vi "program seq..vi"(6 "IOList":T3, 7 "Cluster data":T5, 11 "Filepath":path=path "E:/My Project/2018-2019/Under development/Minda Ind. Switch -ID 144-145/Project/data/trail pro -12.txt") -> (0 "Error Out":errorcluster)   [LabVIEW 2015]
uses:
  Control PB/Active.ctl
  Control PB/deactive.ctl
  Control PB/output control.ctl
  Control PB/input control.ctl
  Control PB/timer.ctl
  Control PB/Remove list.ctl
  Control Button/Exit.ctl
  Control PB/Add_s.ctl
  Control PB/Delete_.ctl
  Control Button/Save.ctl
  Control PB/motor.ctl
  Control PB/Camera.ctl
  Control PB/Barcode.ctl
  Galobal variable_TI.vi
panel:
  out "Step List 4":string[](array[string])
  out "Step List 3":string[](array[string])
  in  "Barcode":T1
  in  "Camera":T2
  out "x <= y?":bool
  out "Cancel":bool
  out "Step List 2":string[](array[string])
  out "Pokayoka Result":cluster{"Sensor Name":string, "Boolean":bool}[](array[cluster])
  in  "Feed Back Channel":i32[](listbox)=[0]
  out "Input":bool[](array[boolean])
  out "Feature List (Out) 2":T4(array[cluster])
  out "error out 2":errorcluster
  in  "Control":bool
  out "Station No":string
  out "Model Name":string
  out "Machine Name":string
  in  "Motor":T6
  in  "Feature List":i32(listbox) caption="Steps List"
  in  "Deletefeature list":T7
  in  "Add feature list":T8
  in  "Deactive":T9
  in  "Active":T10
  in  "Program step":i32(listbox)
  in  "Remove Step":T11
  in  "Wait Time":u32=100 caption="Timer(ms)" max=600000 step=1
  in  "Timer":T12
  in  "Save":T13
  in  "stop":T14
  in  "op Add":T15
  in  "Input Add":T16
  out "Step List":string[](array[string])
  out "output cluster":T17
  in  "Analog":bool
  in  "Analog Input":i32[](listbox)=[0]
  in  "Control Channel":i32[](listbox)=[7]
  in  "Steps":T18(array[cluster])
  in  "Program mode":string="Data"
  out "error out":errorcluster
  out "Feature List (Out)":T19(array[cluster])
  # "Program Sequence Window"
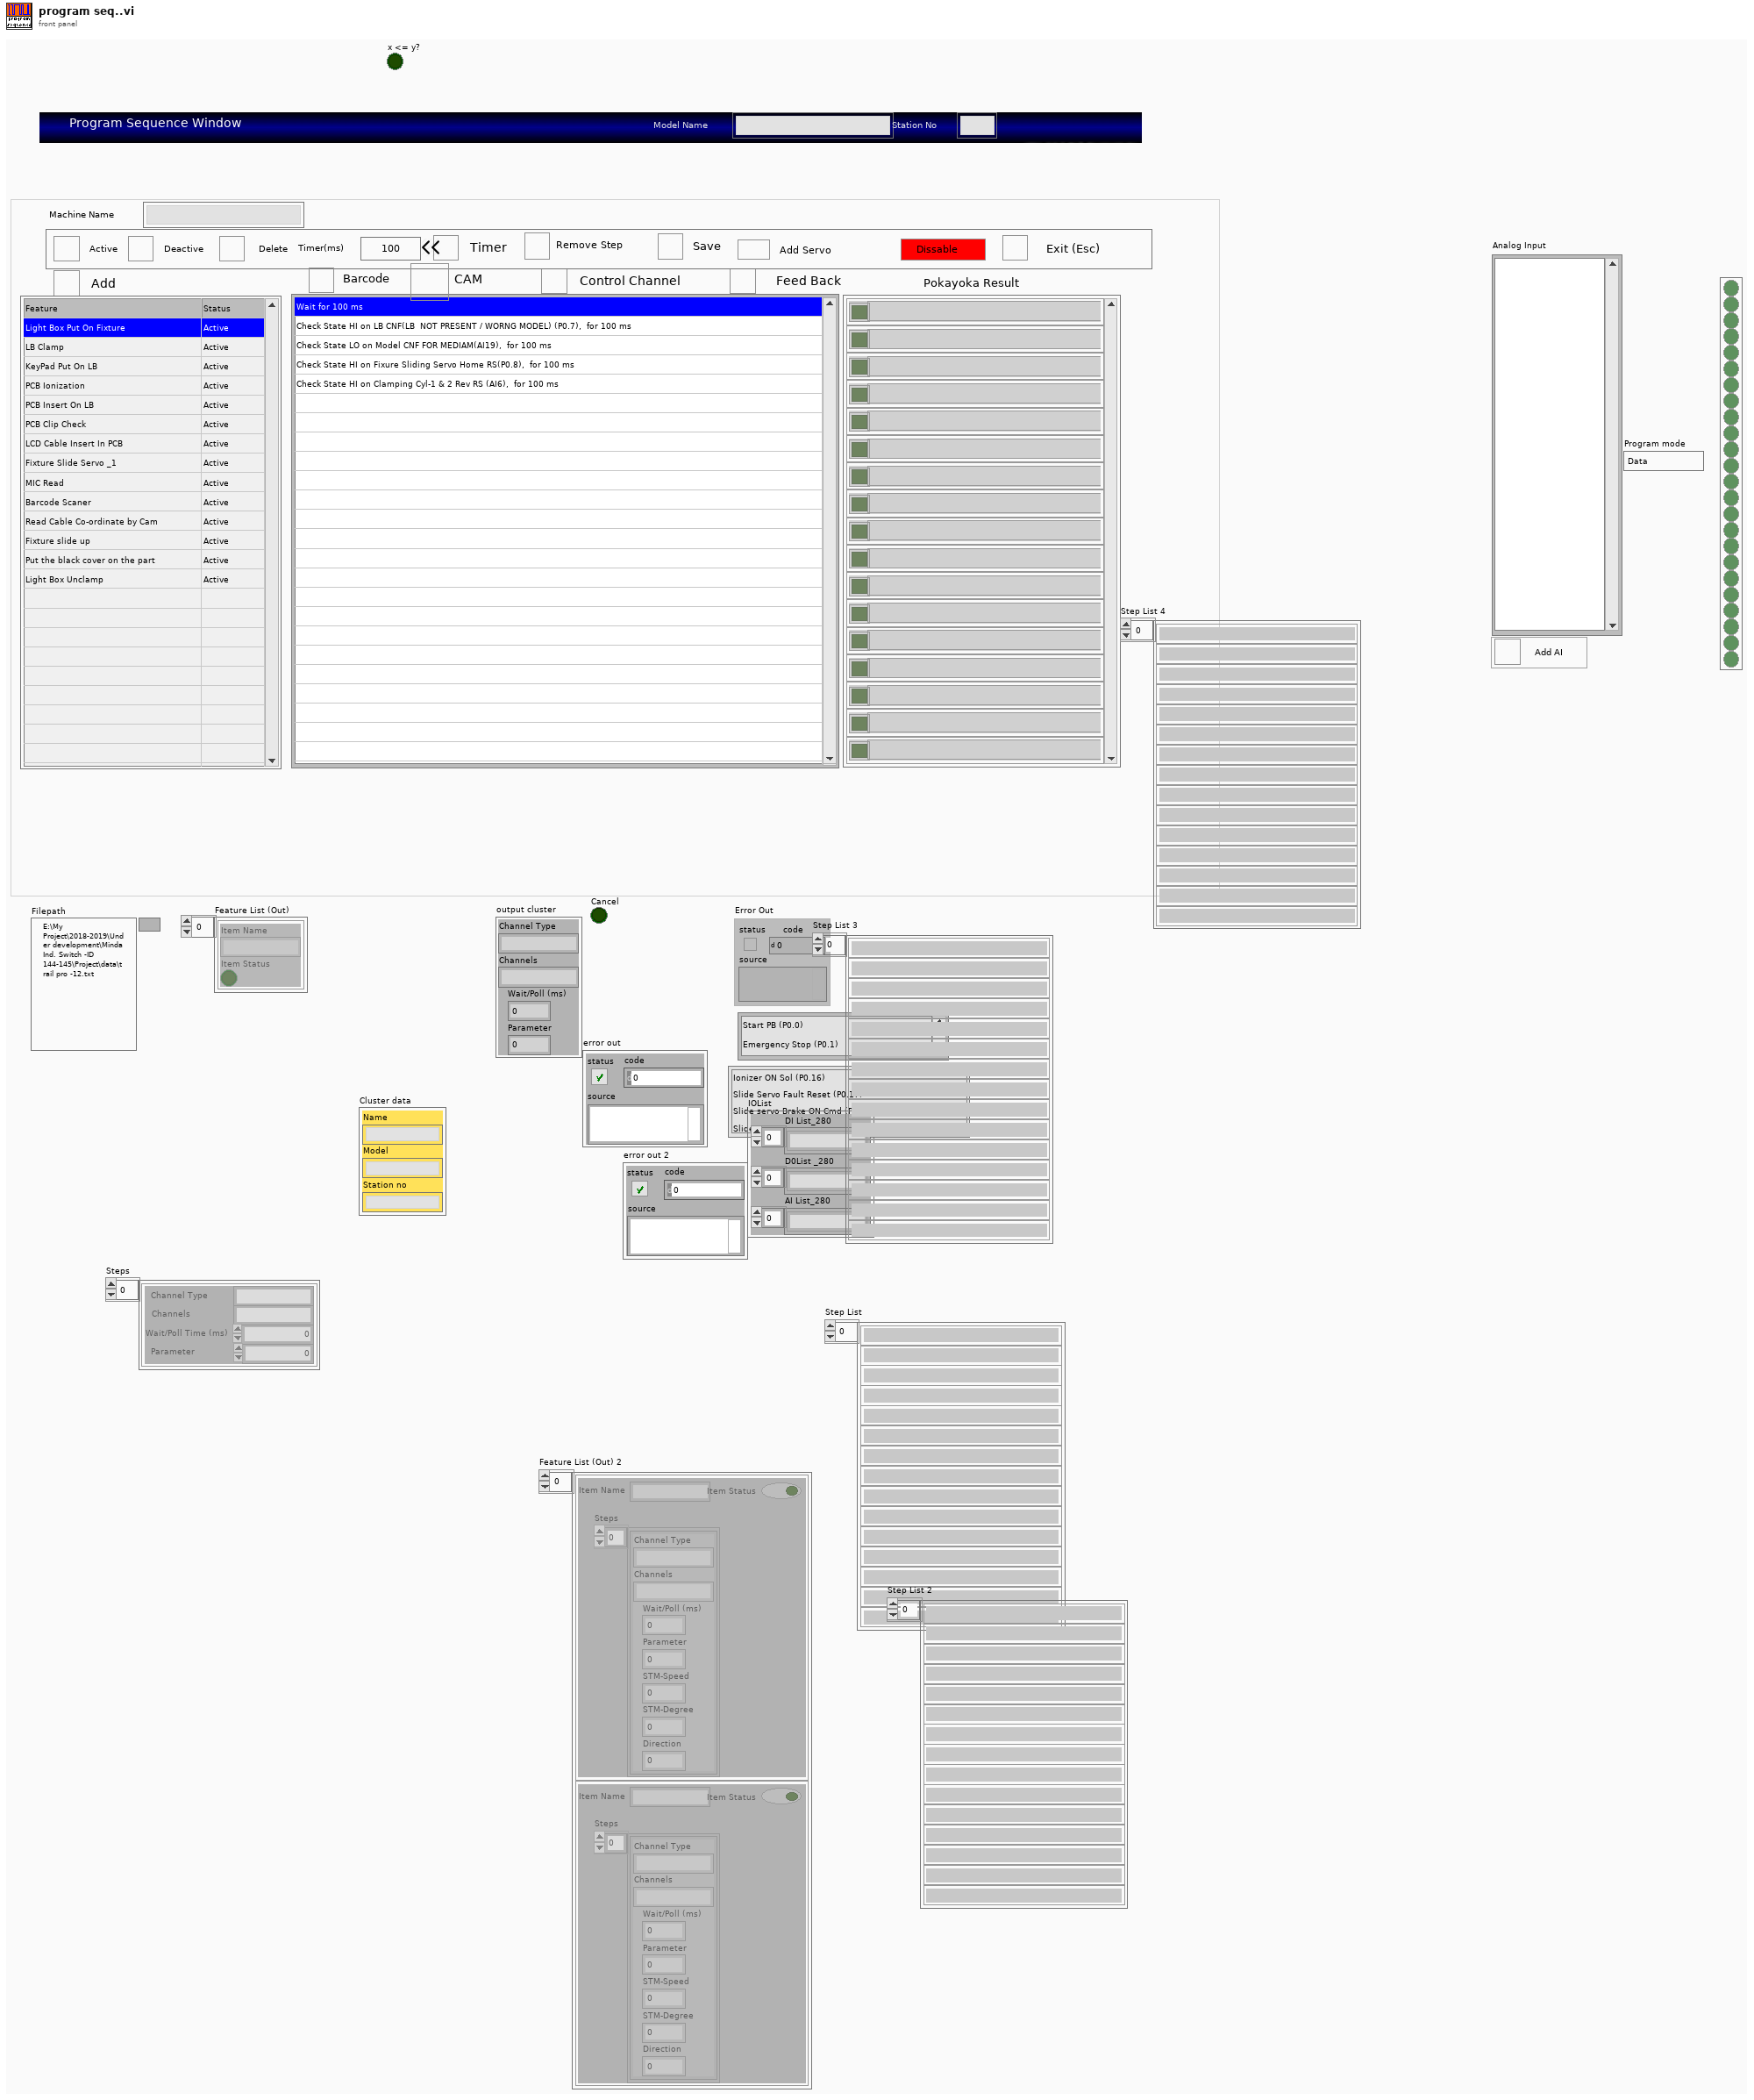
[diagram p1: front panel]
types:
  T1 = typedef "Barcode.ctl" = bool
  T2 = typedef "Camera.ctl" = bool
  T3 = cluster{"DI List_280":string[], "D0List _280":string[], "AI List_280":string[]}
  T4 = cluster{"Item Name":string, "Item Status":bool, "Steps":cluster{"Channel Type":string, "Channels":string, "Wait/Poll (ms)":u32, "Parameter":u8, "STM-Speed":i32, "STM-Degree":u32, "Direction":u8}[]}[]
  T5 = cluster{"Name":string, "Model":string, "Station no":string}
  T6 = typedef "motor.ctl" = bool
  T7 = typedef "Delete_.ctl" = bool
  T8 = typedef "Add_s.ctl" = bool
  T9 = typedef "deactive.ctl" = bool
  T10 = typedef "Active.ctl" = bool
  T11 = typedef "Remove list.ctl" = bool
  T12 = typedef "timer.ctl" = bool
  T13 = typedef "Save.ctl" = bool
  T14 = typedef "Exit.ctl" = bool
  T15 = typedef "output control.ctl" = bool
  T16 = typedef "input control.ctl" = bool
  T17 = cluster{"Channel Type":string, "Channels":string, "Wait/Poll (ms)":u32, "Parameter":u8}
  T18 = cluster{"Channel Type":string, "Channels":string, "Wait/Poll Time (ms)":u32, "Parameter":u8}[]
  T19 = cluster{"Item Name":string, "Item Status":bool}[]
  T20 = cluster{"Channel Type":string, "Channels":string, "Wait/Poll (ms)":u32, "Parameter":u8, "STM-Speed":i32, "STM-Degree":i32, "Direction":u8}
  T21 = cluster{"Item Name":string, "Item Status":bool, "Steps":cluster{"Channel Type":string, "Channels":string, "Wait/Poll (ms)":u32, "Parameter":u8, "STM-Speed":i32, "STM-Degree":u32, "Direction":u8}[]}
  T22 = cluster{"Channel Type":string, "Channels":string, "Wait/Poll (ms)":u32, "Parameter":u8, "STM-Speed":i32, "STM-Degree":u32, "Direction":u8}[]
  T23 = cluster{"Item Name":string, "Active":T10, "Steps":cluster{"Channel Type":string, "Channels":string, "Wait/Poll (ms)":u32, "Parameter":u8, "STM-Speed":i32, "STM-Degree":u32, "Direction":u8}[]}
  T24 = cluster{"Channel Type":string, "Channels":string, "Wait/Poll (ms)":u32, "Parameter":u8, "STM-Speed":i32, "STM-Degree":i32, "Direction":u8}[]
  T25 = cluster{"Feature name ":string, bool, cluster{"Channel Type":string, "Channels":string, "Wait/Poll (ms)":u32, "Parameter":u8, "STM-Speed":i32, "STM-Degree":i32, "Direction":u8}[]}
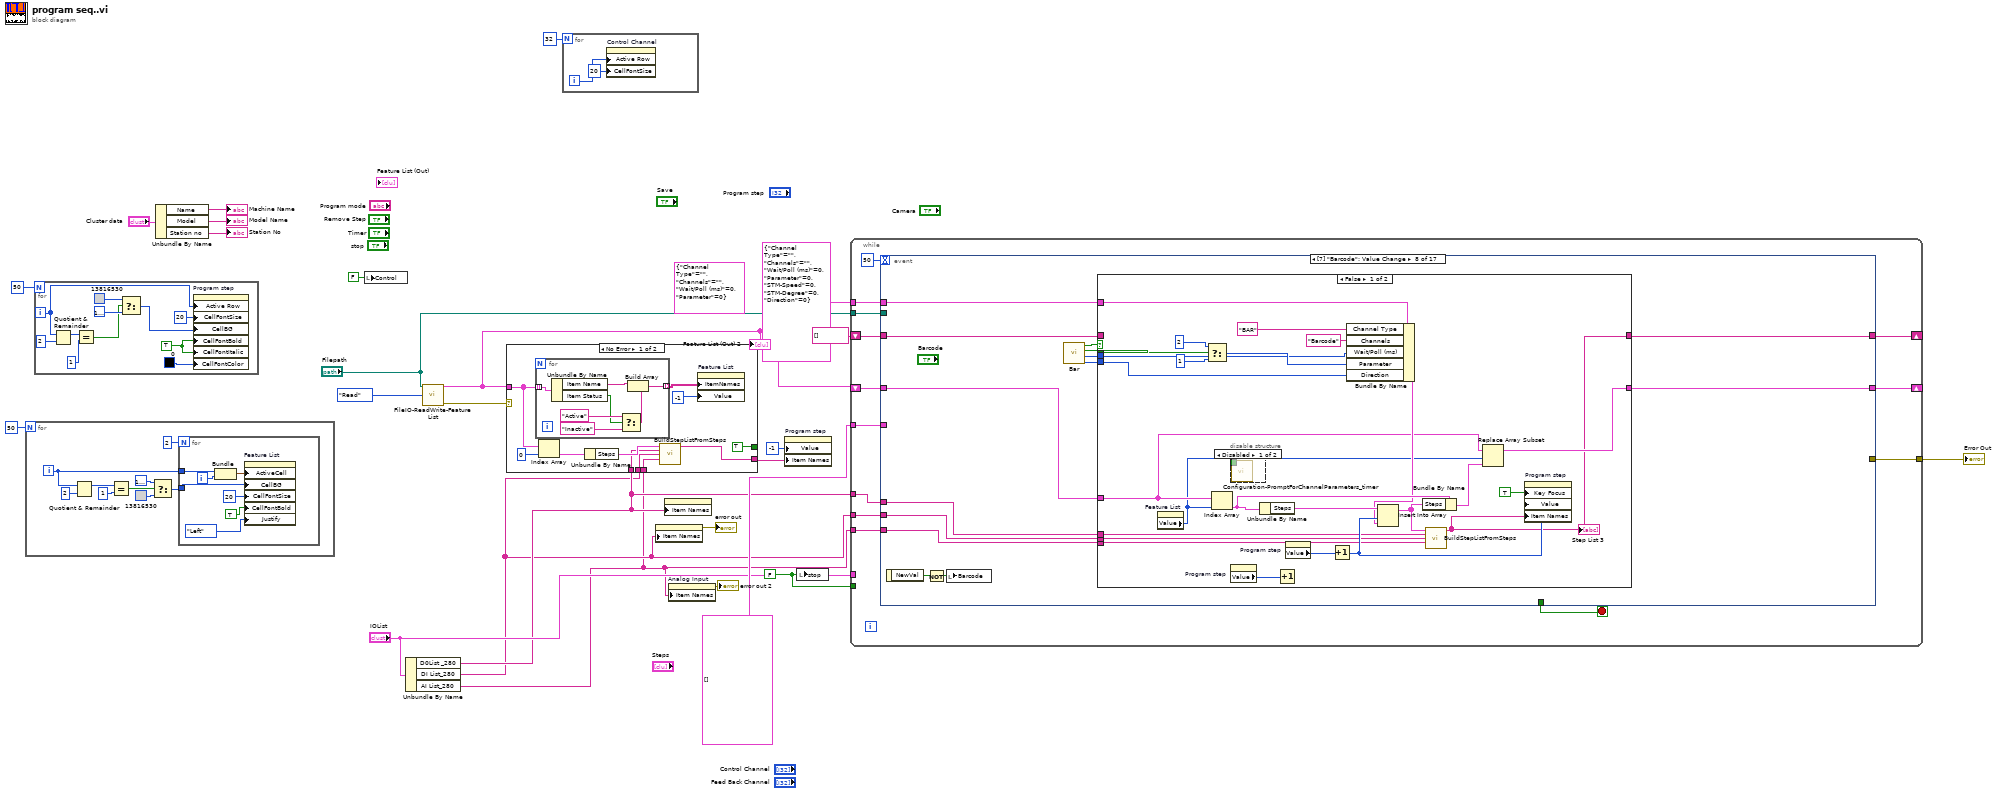
[diagram p0: block diagram]
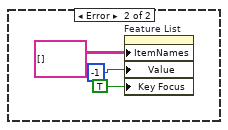
[diagram p2: hidden frame]
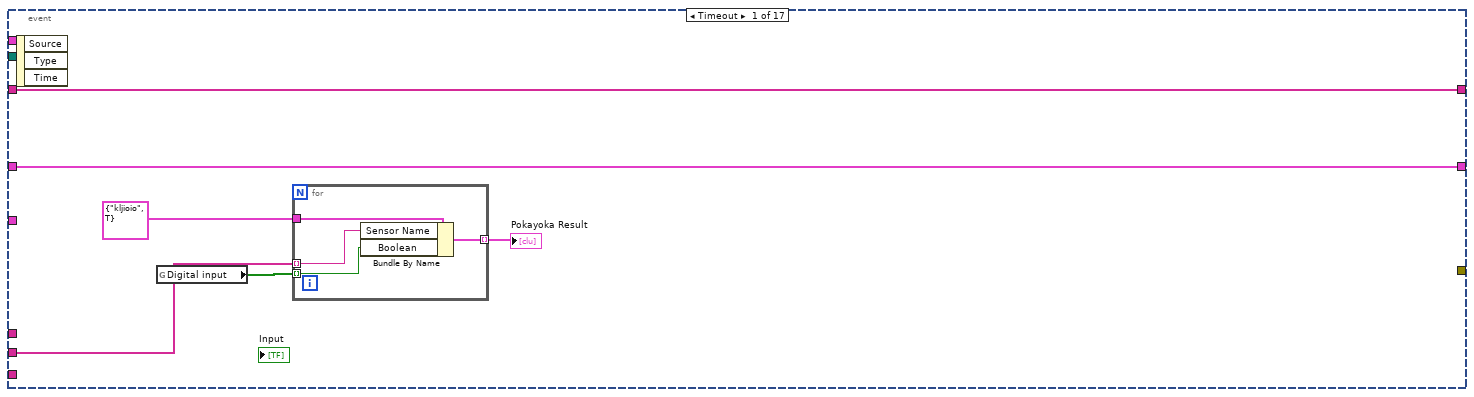
[diagram p3: hidden frame]
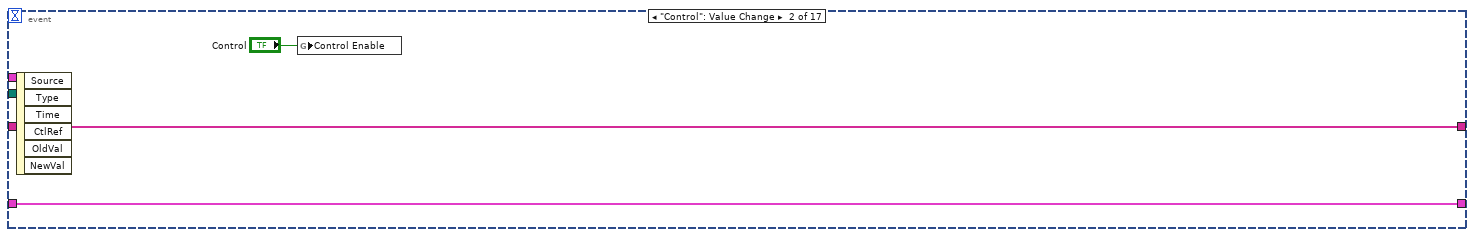
[diagram p4: hidden frame]
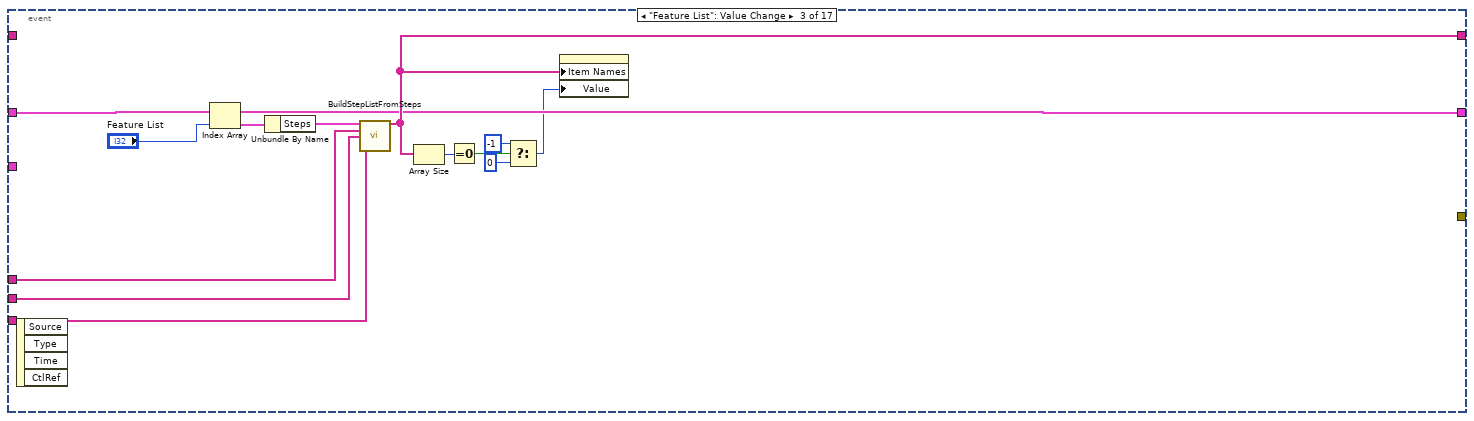
[diagram p5: hidden frame]
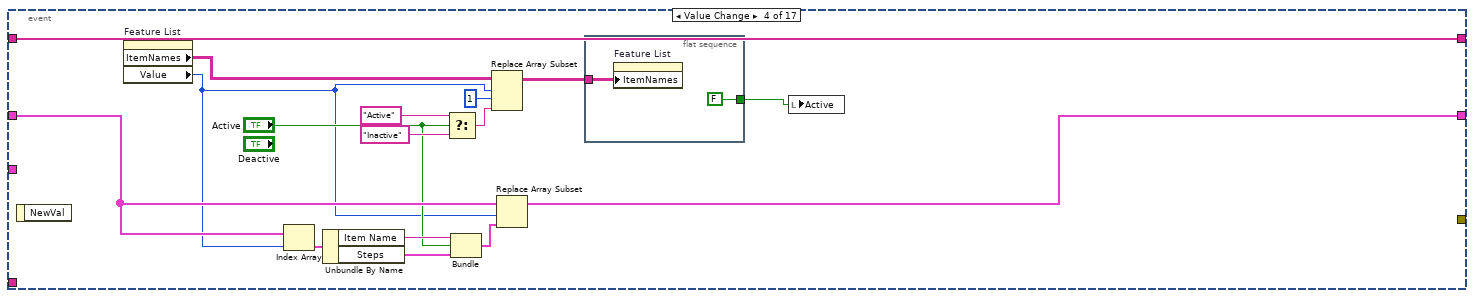
[diagram p6: hidden frame]
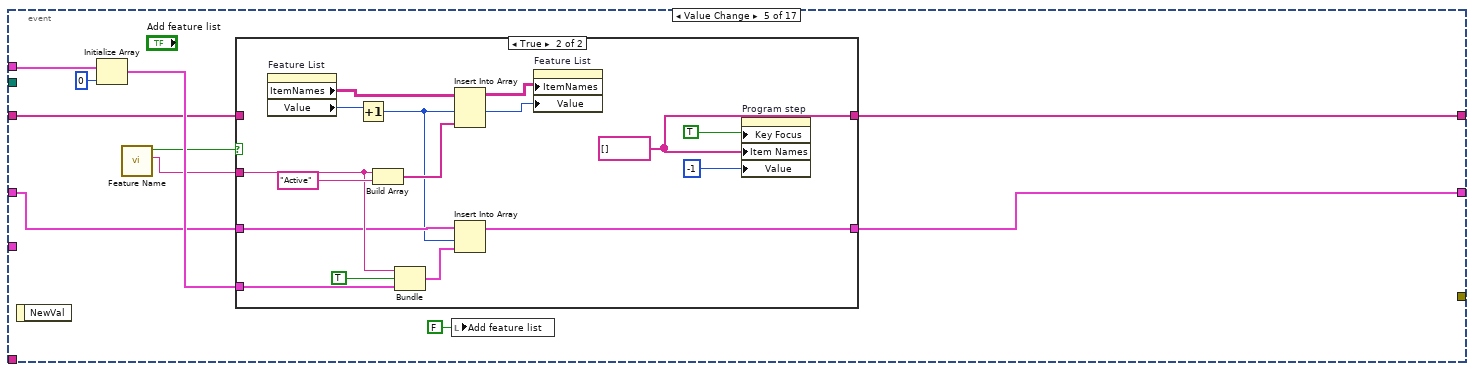
[diagram p7: hidden frame]
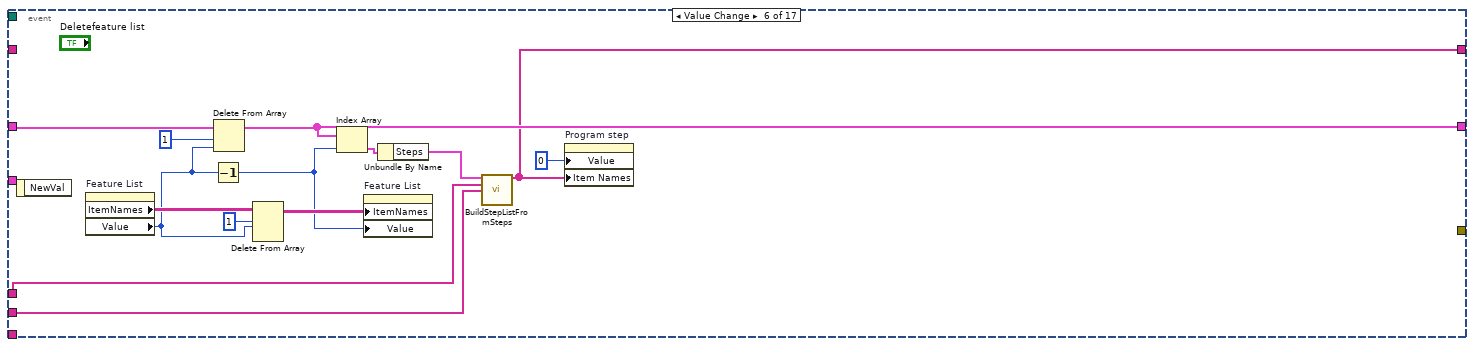
[diagram p9: hidden frame]
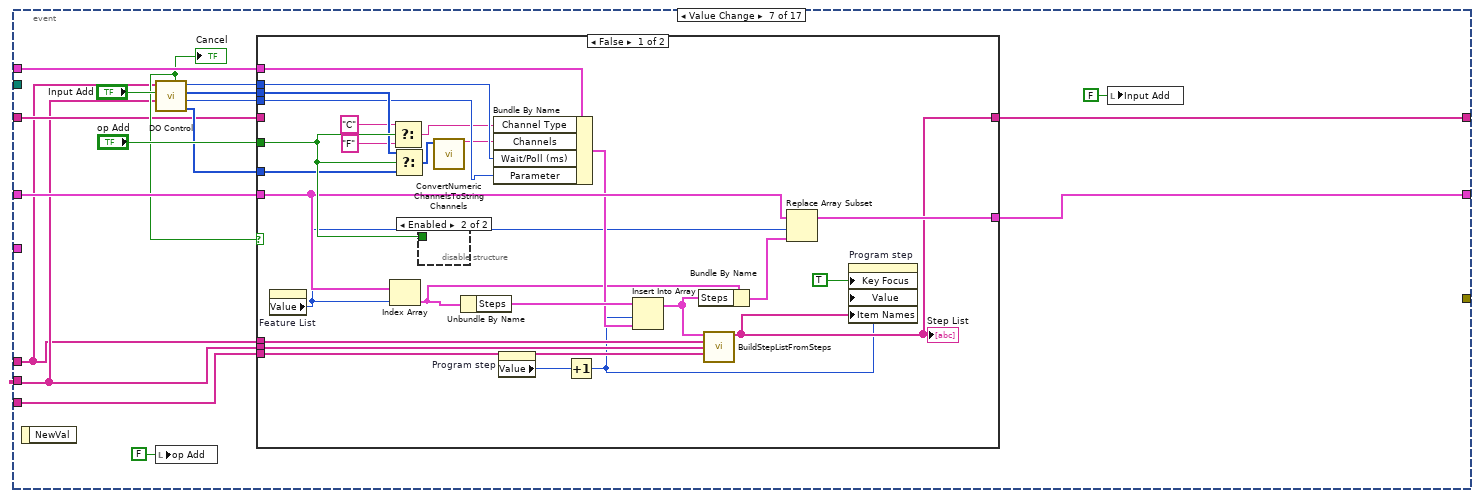
[diagram p10: hidden frame]
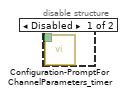
[diagram p11: hidden frame]
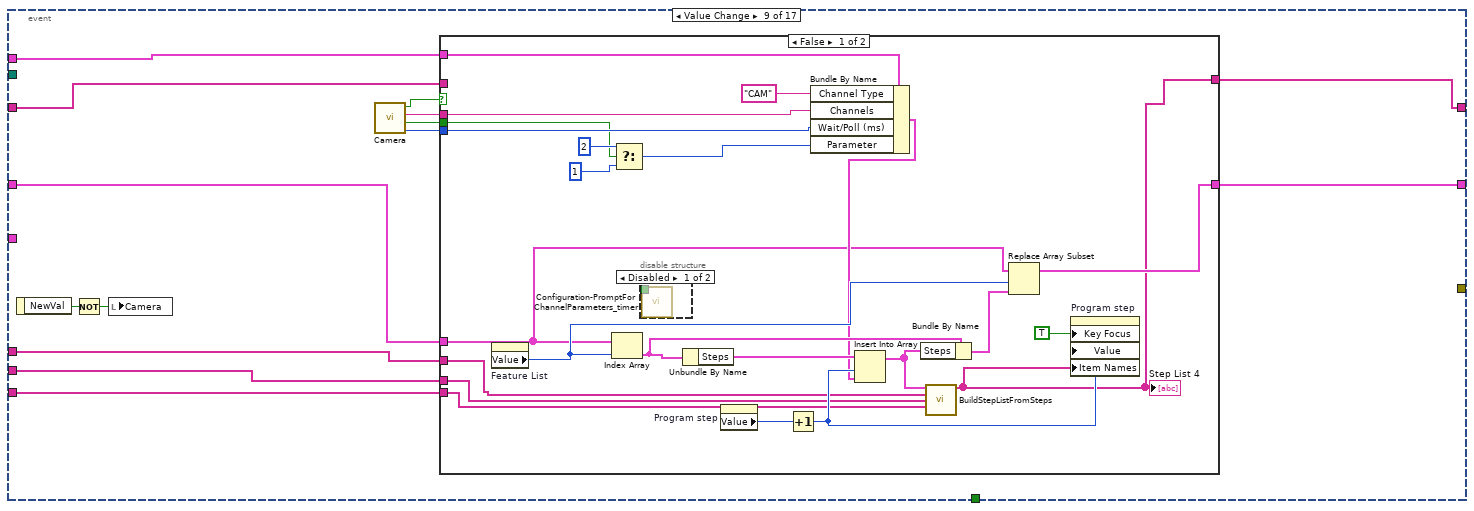
[diagram p15: hidden frame]
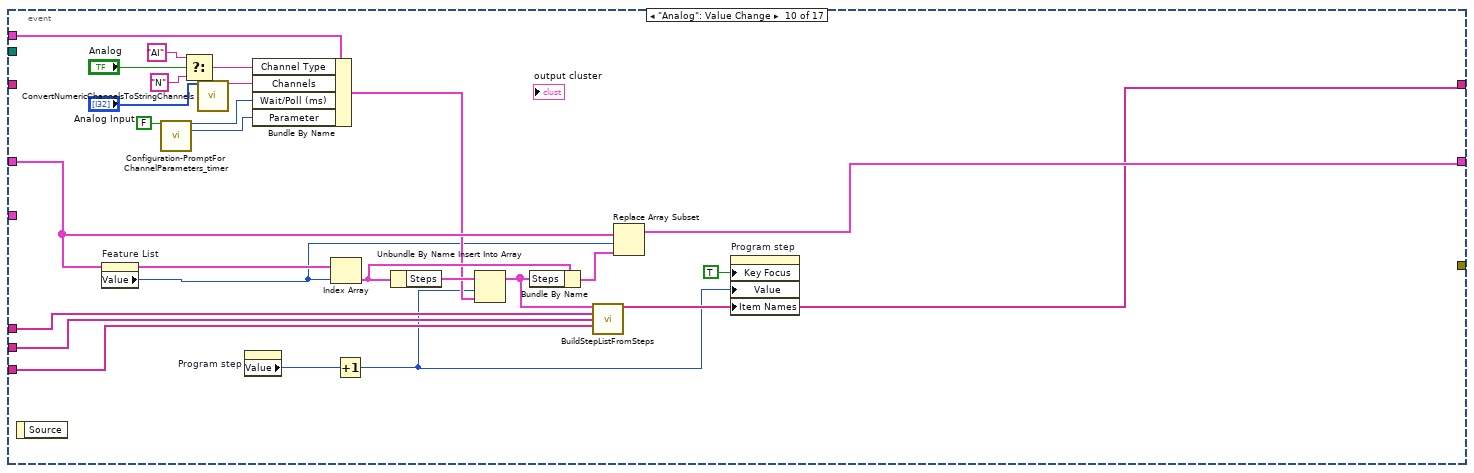
[diagram p18: hidden frame]
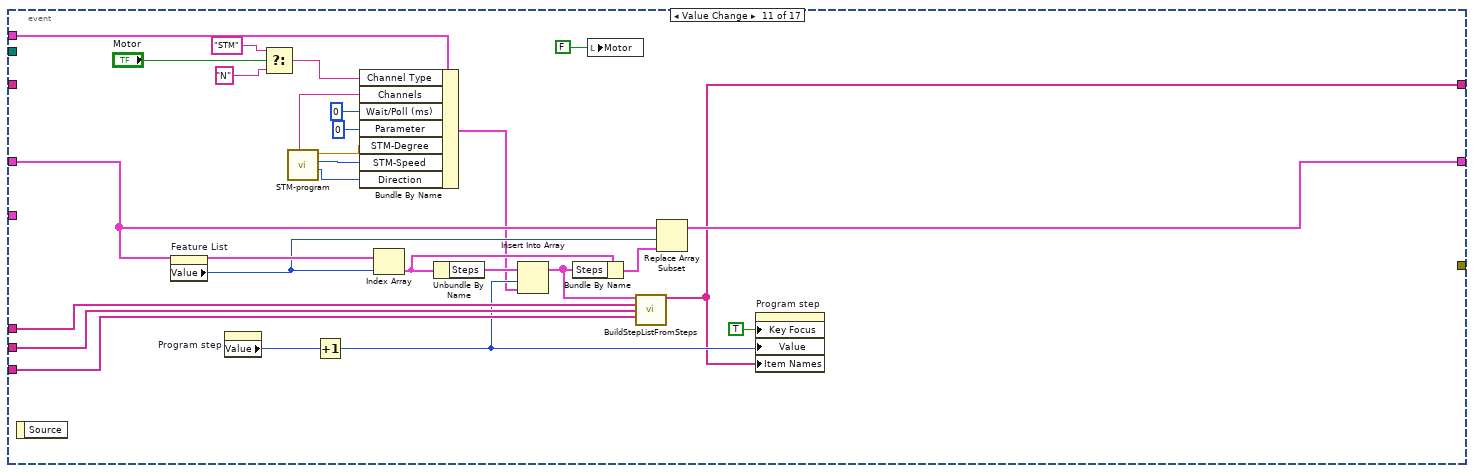
[diagram p19: hidden frame]
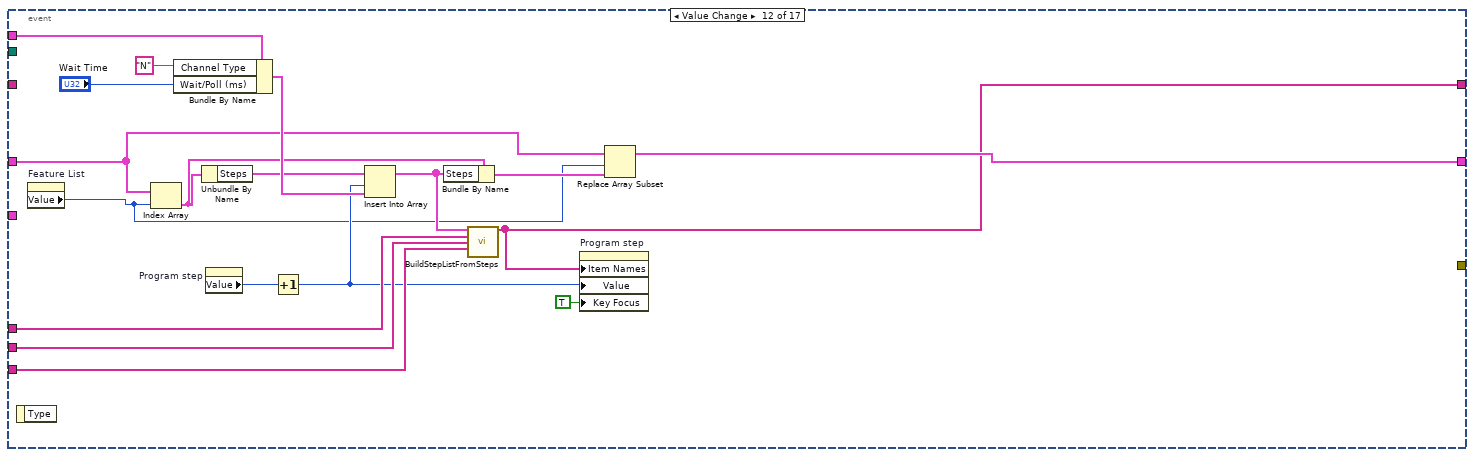
[diagram p20: hidden frame]
diagram:
  w8 = FALSE ("stop")
  (unwired) T17 {"Channel Type"="", "Channels"="", "Wait/Poll (ms)"=0, "Parameter"=0} ("Step")
  n1 = for {
    N: 50 -> [_]
    i -> [w33]
    n2 = Quotient & Remainder(x=w33, y=2) -> (x-y*floor(x/y)=w31:i32)  [unwired: 1 out]
    n3 = Equal?(x=w31, y=1) -> (x = y?=w29:bool)
    n4 = Select(t=u32 16777225 ("Color Box"), s=w29, f=u32 13816530 ("Color Box")) -> (s? t:f=w26:u32)
    n5 = for {
      N: 2 -> [_]
      tunnel: w33 -> [w41]
      tunnel: w26 -> [w38]
      i -> [w40]
      n6 = Bundle(w41, w40) -> (w39:cluster{i32, i32})  [unwired: 1 in]
      n7 = property on="Feature List" class="MCListbox (strict)"("ActiveCell"=w39, "CellBG"=w38, "CellFontSize"=u32 20 ("Active Cell:Cell Font:Size"), "CellFontBold"=TRUE ("Active Cell:Cell Font:Bold"), "Justify"=enum16{"Left", "Center", "Right"}."Left" ("Active Cell:Cell Justification")) -> ()  [unwired: 2 in, 2 out]
    }
  }
  n8 = for {
    N: 50 -> [_]
    i -> [w46]
    w43 = TRUE
    n9 = Quotient & Remainder(x=w46, y=2) -> (x-y*floor(x/y)=w49:i32)  [unwired: 1 out]
    n10 = Equal?(x=w49, y=1) -> (x = y?=w47:bool)
    n11 = Select(t=u32 13816530 ("Color Box"), s=w47, f=u32 16777226 ("Color Box")) -> (s? t:f=w44:u32)
    n12 = property on="Program step" class="LstBox (strict)"("Active Row"=w46, "CellFontSize"=u32 20 ("Active Row:Cell Font:Size"), "CellBG"=w44, "CellFontBold"=w43, "CellFontItalic"=w43, "CellFontColor"=u32 0 ("Color Box")) -> ()  [unwired: 2 in, 2 out]
  }
  n13 = Unbundle By Name("Cluster data") -> ("Name"=→"Machine Name":string, "Model"=→"Model Name":string, "Station no"=→"Station No":string)
  n14 = local write "Control"(FALSE ("Control")) -> ()
  n15 = Unbundle By Name("IOList") -> ("D0List _280"=w4:string[], "DI List_280"=w3:string[], "AI List_280"=w2:string[])
  n16 = call "FileIO-ReadWrite-FeatureList.vi"("Filepath"="Filepath", "Read/Write"=enum16{"Read", "Write"}."Read") -> ("Feature List (Out)"=w16:T4, "Error Out"=w20:errorcluster)  [unwired: 12 in]
  "Feature List (Out) 2" <- w16
  n17 = case shown="No Error" w20 {
    tunnel: w16 -> [w63 _]
    tunnel: w4 -> [w59 _]
    tunnel: w3 -> [w58 _]
    tunnel: w2 -> [w57 _]
    tunnel: [w56 _] -> w19
    tunnel: [TRUE ("Key Focus") _] -> _
    frame No Error {
      n18 = for {
        tunnel: w63 -> [w70] mode=indexing
        tunnel: [w64] -> w54 mode=indexing
        n19 = Unbundle By Name(w70) -> ("Item Name"=w66:string, "Item Status"=w67:bool)
        n20 = Select(t="Active", s=w67, f="Inactive") -> (s? t:f=w65:string)
        n21 = Build Array(w66, w65) -> (w64:string[])
      }
      n22 = Index Array(array=w63, index=0) -> (element=w61:T21)
      n23 = Unbundle By Name(w61) -> ("Steps"=w60:T22)
      n24 = call "BuildStepListFromSteps.vi"("Steps"=w60, "Control Channels"=w59, "Feedback Channels"=w58, "AI"=w57) -> ("Step List"=w56:string[])  [unwired: 11 in]
      n25 = property on="Feature List" class="MCListbox (strict)"("ItemNames"=w54, "Value"=-1 ("Feautre list")) -> ()  [unwired: 2 in, 2 out]
    }
    frame Error {
      n26 = property on="Feature List" class="MCListbox (strict)"("ItemNames"=string[][] [] ("Item Names"), "Value"=-1 ("Feautre list"), "Key Focus"=TRUE) -> ()  [unwired: 2 in, 2 out]
    }
  }
  n27 = for {
    N: 32 -> [_]
    i -> [w75]
    n28 = property on="Control Channel" class="LstBox (strict)"("Active Row"=w75, "CellFontSize"=u32 20 ("Active Row:Cell Font:Size")) -> ()  [unwired: 2 in, 2 out]
  }
  n29 = property on="Feed Back Channel" class="LstBox (strict)"("Item Names"=w3) -> (error out=→"error out":errorcluster)  [unwired: 2 in, 1 out]
  n30 = property on="Control Channel" class="LstBox (strict)"("Item Names"=w4) -> ()  [unwired: 2 in, 2 out]
  n31 = property on="Analog Input" class="LstBox (strict)"("Item Names"=w2) -> (error out=→"error out 2":errorcluster)  [unwired: 2 in, 1 out]
  n32 = property on="Program step" class="LstBox (strict)"("Value"=-1 ("Step feautre list"), "Item Names"=w19) -> ()  [unwired: 2 in, 2 out]
  n33 = local write "stop"(w8) -> ()
  n34 = while {
    shift-right: [w86] -> _
    shift-left: w16 -> [w77]
    tunnel: T20 {"Channel Type"="", "Channels"="", "Wait/Poll (ms)"=0, "Parameter"=0, "STM-Speed"=0, "STM-Degree"=0, "Direction"=0} ("Step") -> [w87]
    shift-right: [w85] -> _
    shift-left: string[] [] ("Step List") -> [w84]
    tunnel: w4 -> [w83]
    tunnel: w3 -> [w82]
    tunnel: [w81] -> w23
    tunnel: w2 -> [w80]
    tunnel: T4 [] ("Feature List (Out) 2") -> [w79]
    tunnel: "Filepath" -> [w78]
    tunnel: w8 -> [_]
    tunnel: "IOList" -> [_]
    stop <- w88 stop-if-true
    n35 = event shown="[7] \"Barcode\": Value Change" {
      selector: _ -> [_ _ _ _ _ _ _ _ _ _ _ _ _ _ _ _ _]
      dyn-events: _ -> [_ _ _ _ _ _ _ _ _ _ _ _ _ _ _ _ _]
      timeout: 50 -> [_ _ _ _ _ _ _ _ _ _ _ _ _ _ _ _ _]
      tunnel: [_ _ _ _ _ _ _ _ _ _ _ _ _ _ TRUE ("stop") _ TRUE ("Discard?")] -> w88
      tunnel: w77 -> [w94 w100 w105 w122 w139 w171 w187 w228 w271 w311 w341 w362 w384 w393 w453 w475 w552]
      tunnel: w87 -> [_ _ _ _ w142 _ w190 w233 w275 w318 w346 w371 _ _ _ w476 _]
      tunnel: [w94 w100 w105 w120 w138 w170 w188 w227 w270 w306 w333 w361 w383 w395 w453 w471 w552] -> w86
      tunnel: [w93 w101 w108 w119 w135 w165 w186 w226 w269 w305 w332 w358 w378 w410 w452 w470 w553] -> w85
      tunnel: w84 -> [w93 w101 _ w119 w134 _ w177 w221 w265 _ _ _ _ _ w452 w469 w553]
      tunnel: w83 -> [_ _ w107 _ _ w167 w175 w229 w272 w308 w338 w360 w380 w412 _ w472 _]
      tunnel: w82 -> [w92 _ w106 _ _ w166 w176 w230 w273 w309 w337 w359 w379 w411 _ w473 _]
      tunnel: [_ _ _ _ _ _ _ _ _ _ _ _ _ w403 _ _ _] -> w81
      tunnel: w80 -> [_ _ w104 _ _ _ w185 w231 w274 w310 w336 w357 _ w404 _ w474 _]
      tunnel: w79 -> [_ _ _ _ _ _ _ _ _ _ _ _ _ w409 _ _ _]
      tunnel: w78 -> [_ _ _ _ _ _ _ _ _ _ _ _ _ w394 _ _ _]
      event Timeout {
        n36 = event-data() -> ()  [unwired: 1 in, 3 out]
        n37 = global read "Galobal variable_TI.vi" "Digital input"() -> (w89:bool[])
        n38 = for {
          tunnel: w92 -> [w97] mode=indexing
          tunnel: cluster{"Sensor Name":string, "Boolean":bool} {"Sensor Name"="kljioio", "Boolean"=TRUE} ("Cluster") -> [w98]
          tunnel: [w96] -> w90 mode=indexing
          tunnel: w89 -> [w95] mode=indexing
          n39 = Bundle By Name(cluster=w98, "Sensor Name"=w97, "Boolean"=w95) -> (w96:cluster{"Sensor Name":string, "Boolean":bool})
        }
        "Pokayoka Result" <- w90
      }
      event "Control": Value Change {
        n40 = event-data() -> ()  [unwired: 1 in, 6 out]
        n41 = global write "Galobal variable_TI.vi" "Control Enable"("Control") -> ()
      }
      event "Feature List": Value Change {
        n42 = event-data() -> ()  [unwired: 1 in, 4 out]
        n43 = Index Array(array=w105, index="Feature List") -> (element=w114:T21)
        n44 = Unbundle By Name(w114) -> ("Steps"=w113:T22)
        n45 = call "BuildStepListFromSteps.vi"("Steps"=w113, "Control Channels"=w107, "Feedback Channels"=w106, "AI"=w104) -> ("Step List"=w108:string[])  [unwired: 11 in]
        n46 = Array Size(array=w108) -> (size(s)=w110:i32)
        n47 = Equal To 0?(x=w110) -> (x = 0?=w112:bool)
        n48 = Select(t=-1 ("Step List"), s=w112, f=0 ("Step List")) -> (s? t:f=w103:i32)
        n49 = property on="Program step" class="LstBox (strict)"("Item Names"=w108, "Value"=w103) -> ()  [unwired: 2 in, 2 out]
      }
      event Value Change {
        n50 = event-data() -> ()  [unwired: 1 in, 1 out]
        n51 = property on="Feature List" class="MCListbox (strict)"() -> ("ItemNames"=w118:string[][], "Value"=w116:i32)  [unwired: 2 in, 2 out]
        n52 = Index Array(array=w122, index=w116) -> (element=w128:T21)
        n53 = Unbundle By Name(w128) -> ("Item Name"=w129:string, "Steps"=w130:T22)
        n54 = Select(t="Active", s="Active", f="Inactive" ("element")) -> (s? t:f=w125:string)
        n55 = Bundle("Item Name"=w129, "Active"="Active", "Steps"=w130) -> (w127:T23)  [unwired: 1 in]
        n56 = Replace Array Subset(array=w118, new element=w125, index (row)=w116, index (col)=1 ("disabled index (col)")) -> (w117:string[][])
        n57 = Replace Array Subset(array=w122, new element=w127, index=w116) -> (w120:T4)
        n58 = flat-sequence {
          tunnel: w117 -> [w132]
          tunnel: [T10 FALSE ("Active")] -> w115
          frame #0 {
            n59 = property on="Feature List" class="MCListbox (strict)"("ItemNames"=w132) -> ()  [unwired: 2 in, 2 out]
          }
        }
        n60 = local write "Active"(w115) -> ()
      }
      event Value Change {
        n61 = event-data() -> ()  [unwired: 1 in, 1 out]
        n62 = Initialize Array(w142, 0 ("dimension size")) -> (w140:T24)
        n63 = call "Feature Name.vi"() -> ("Feature name"=w136:string, "Out"=w137:bool)  [unwired: 10 in]
        n64 = case shown="True" w137 {
          tunnel: w140 -> [_ w158]
          tunnel: w139 -> [w144 w153]
          tunnel: [w144 w155] -> w138
          tunnel: w136 -> [_ w154]
          tunnel: [w143 w151] -> w135
          tunnel: w134 -> [w143 _]
          frame False {
          }
          frame True {
            w151 = string[] [] ("Item Names")
            n65 = property on="Feature List" class="MCListbox (strict)"() -> ("ItemNames"=w148:string[][], "Value"=w145:i32)  [unwired: 2 in, 2 out]
            n66 = Increment(x=w145) -> (x+1=w146:i32)
            n67 = Build Array(w154, "Active") -> (w149:string[])
            n68 = Bundle("Feature name"=w154, TRUE, w158) -> (w156:T25)  [unwired: 1 in]
            n69 = Insert Into Array(array=w148, index (row)=w146, new element=w149) -> (w147:string[][])  [unwired: 1 in]
            n70 = Insert Into Array(array=w153, index=w146, new element=w156) -> (w155:T4)
            n71 = property on="Feature List" class="MCListbox (strict)"("ItemNames"=w147, "Value"=w146) -> ()  [unwired: 2 in, 2 out]
            n72 = property on="Program step" class="LstBox (strict)"("Key Focus"=TRUE, "Item Names"=w151, "Value"=-1 ("Step feautre list")) -> ()  [unwired: 2 in, 2 out]
          }
        }
        n73 = local write "Add feature list"(FALSE ("Add feature list")) -> ()
      }
      event Value Change {
        n74 = event-data() -> ()  [unwired: 1 in, 1 out]
        n75 = property on="Feature List" class="MCListbox (strict)"() -> ("ItemNames"=w163:string[][], "Value"=w162:i32)  [unwired: 2 in, 2 out]
        n76 = Decrement(x=w162) -> (x-1=w160:i32)
        n77 = Delete From Array(array=w171, length=1, index=w162) -> (array with subset deleted=w170:T4)  [unwired: 1 out]
        n78 = Delete From Array(array=w163, length=1, index (row)=w162) -> (array with subset deleted=w161:string[][])  [unwired: 1 in, 1 out]
        n79 = Index Array(array=w170, index=w160) -> (element=w169:T21)
        n80 = property on="Feature List" class="MCListbox (strict)"("ItemNames"=w161, "Value"=w160) -> ()  [unwired: 2 in, 2 out]
        n81 = Unbundle By Name(w169) -> ("Steps"=w168:T22)
        n82 = call "BuildStepListFromSteps.vi"("Steps"=w168, "Control Channels"=w167, "Feedback Channels"=w166) -> ("Step List"=w165:string[])  [unwired: 12 in]
        n83 = property on="Program step" class="LstBox (strict)"("Value"=0 ("Step feautre list"), "Item Names"=w165) -> ()  [unwired: 2 in, 2 out]
      }
      event Value Change {
        n84 = event-data() -> ()  [unwired: 1 in, 1 out]
        n85 = call "DO Control.vi"("DI List_280"=w176, "s"="Input Add", "Control"=w175) -> ("Feedback"=w180:i32[], "Parameter (Out)"=w182:u8, "Control Channel"=w184:i32[], "Poll Time (Out)"=w183:u32, "Cancel"=w178:bool)  [unwired: 3 in, 1 out]
        "Cancel" <- w178
        n86 = local write "op Add"(T15 FALSE ("op Add")) -> ()
        n87 = case shown="False" w178 {
          tunnel: w190 -> [w216 _]
          tunnel: "op Add" -> [w215 _]
          tunnel: [w214 w219] -> w188
          tunnel: w187 -> [w213 w219]
          tunnel: w175 -> [w212 _]
          tunnel: w176 -> [w211 _]
          tunnel: [w210 w218] -> w186
          tunnel: w185 -> [w209 _]
          tunnel: w184 -> [w208 _]
          tunnel: w183 -> [w207 _]
          tunnel: w182 -> [w206 _]
          tunnel: w180 -> [w205 _]
          tunnel: w177 -> [_ w218]
          frame False {
            n88 = property on="Feature List" class="MCListbox (strict)"() -> ("Value"=w191:i32)  [unwired: 2 in, 2 out]
            n89 = Index Array(array=w213, index=w191) -> (element=w197:T21)
            n90 = Select(t="C", s=w215, f="F") -> (s? t:f=w202:string)
            n91 = Select(t=w208, s=w215, f=w205) -> (s? t:f=w201:i32[])
            n92 = disable-structure shown="Enabled" {
              disable-tunnel: w215 -> [w217 _]
              frame Disabled {
                n93 = call "Configuration-PromptForChannelParameters_timer.vi"("Control/Feedback\n(Default: False = Feedback)"=w217) -> ()  [unwired: 13 in, 2 out]
              }
              frame Enabled {
              }
            }
            n94 = call "ConvertNumericChannelsToStringChannels.vi"("Channels (In)"=w201) -> ("Channels (A:B:C:D...) (Out)"=w200:string)  [unwired: 14 in]
            n95 = Unbundle By Name(w197) -> ("Steps"=w199:T22)
            n96 = Bundle By Name(cluster=w216, "Channel Type"=w202, "Channels"=w200, "Wait/Poll (ms)"=w207, "Parameter"=w206) -> (w198:T20)
            n97 = property on="Program step" class="LstBox (strict)"() -> ("Value"=w192:i32)  [unwired: 2 in, 2 out]
            n98 = Increment(x=w192) -> (x+1=w193:i32)
            n99 = Insert Into Array "Insert Into Array"(array=w199, index=w193, new element=w198) -> (w195:T22)
            n100 = Bundle By Name(cluster=w197, "Steps"=w195) -> (w196:T21)
            n101 = call "BuildStepListFromSteps.vi"("Steps"=w195, "Control Channels"=w212, "Feedback Channels"=w211, "AI"=w209) -> ("Step List"=w210:string[])  [unwired: 11 in]
            "Step List" <- w210
            n102 = Replace Array Subset(array=w213, new element=w196, index=w191) -> (w214:T4)
            n103 = property on="Program step" class="LstBox (strict)"("Key Focus"=TRUE, "Value"=w193, "Item Names"=w210) -> ()  [unwired: 2 in, 2 out]
          }
          frame True {
          }
        }
        n104 = local write "Input Add"(T16 FALSE ("Input Add")) -> ()
      }
      event Value Change {
        n105 = event-data() -> ("NewVal"=w224:T1)  [unwired: 1 in]
        n106 = Not(x=w224) -> (.not. x?=w223:T1)
        n107 = local write "Barcode"(w223) -> ()
        n108 = call "Bar.vi"() -> ("Numeric"=w220:i32, "Time Out Value"=w225:u8, "Barcode Scane"=w232:bool, "Out"=w222:bool)  [unwired: 8 in]
        n109 = case shown="False" w222 {
          tunnel: w233 -> [w258 _]
          tunnel: w232 -> [w255 _]
          tunnel: w231 -> [w242 _]
          tunnel: w230 -> [w241 _]
          tunnel: w229 -> [w240 _]
          tunnel: w228 -> [w239 w260]
          tunnel: [w238 w260] -> w227
          tunnel: [w237 w261] -> w226
          tunnel: w225 -> [w236 _]
          tunnel: w221 -> [_ w261]
          tunnel: w220 -> [w234 _]
          frame False {
            n110 = property on="Feature List" class="MCListbox (strict)"() -> ("Value"=w235:i32)  [unwired: 2 in, 2 out]
            n111 = Select(t=2, s=w255, f=1) -> (s? t:f=w252:i32)
            n112 = Index Array(array=w239, index=w235) -> (element=w250:T21)
            n113 = disable-structure shown="Disabled" {
              disable-tunnel: _ -> [w259 _]
              frame Disabled {
                n114 = call "Configuration-PromptForChannelParameters_timer.vi"("Control/Feedback\n(Default: False = Feedback)"=w259) -> ()  [unwired: 13 in, 2 out]
              }
              frame Enabled {
              }
            }
            n115 = property on="Program step" class="LstBox (strict)"() -> ("Value"=w244:i32)  [unwired: 2 in, 2 out]
            n116 = Unbundle By Name(w250) -> ("Steps"=w251:T22)
            n117 = Increment(x=w244) -> ()  [unwired: 1 out]
            n118 = property on="Program step" class="LstBox (strict)"() -> ("Value"=w245:i32)  [unwired: 2 in, 2 out]
            n119 = Increment(x=w245) -> (x+1=w246:i32)
            n120 = Bundle By Name(cluster=w258, "Channel Type"="BAR", "Channels"="Barcode", "Wait/Poll (ms)"=w236, "Parameter"=w252, "Direction"=w234) -> (w243:T20)
            n121 = Insert Into Array "Insert Into Array"(array=w251, index=w246, new element=w243) -> (w248:T22)
            n122 = Bundle By Name(cluster=w250, "Steps"=w248) -> (w249:T21)
            n123 = call "BuildStepListFromSteps.vi"("Steps"=w248, "Control Channels"=w240, "Feedback Channels"=w241, "AI"=w242) -> ("Step List"=w237:string[])  [unwired: 11 in]
            "Step List 3" <- w237
            n124 = Replace Array Subset(array=w239, new element=w249, index=w235) -> (w238:T4)
            n125 = property on="Program step" class="LstBox (strict)"("Key Focus"=TRUE, "Value"=w246, "Item Names"=w237) -> ()  [unwired: 2 in, 2 out]
          }
          frame True {
          }
        }
      }
      event Value Change {
        n126 = event-data() -> ("NewVal"=w262:T2)  [unwired: 1 in]
        n127 = Not(x=w262) -> (.not. x?=w263:T2)
        n128 = local write "Camera"(w263) -> ()
        n129 = call "Camera.vi"() -> ("Time Out (ms) 2"=w267:u8, "Camera 2"=w266:bool, "Feature name"=w268:string, "Out"=w264:bool)  [unwired: 8 in]
        n130 = case shown="False" w264 {
          tunnel: w275 -> [w285 _]
          tunnel: w274 -> [w284 _]
          tunnel: w273 -> [w283 _]
          tunnel: w272 -> [w282 _]
          tunnel: w271 -> [w281 w300]
          tunnel: [w280 w300] -> w270
          tunnel: [w279 w301] -> w269
          tunnel: w268 -> [w278 _]
          tunnel: w267 -> [w277 _]
          tunnel: w266 -> [w276 _]
          tunnel: w265 -> [_ w301]
          frame False {
            n131 = property on="Feature List" class="MCListbox (strict)"() -> ("Value"=w287:i32)  [unwired: 2 in, 2 out]
            n132 = Index Array(array=w281, index=w287) -> (element=w293:T21)
            n133 = Select(t=2, s=w276, f=1) -> (s? t:f=w295:i32)
            n134 = disable-structure shown="Disabled" {
              disable-tunnel: _ -> [w299 _]
              frame Disabled {
                n135 = call "Configuration-PromptForChannelParameters_timer.vi"("Control/Feedback\n(Default: False = Feedback)"=w299) -> ()  [unwired: 13 in, 2 out]
              }
              frame Enabled {
              }
            }
            n136 = Unbundle By Name(w293) -> ("Steps"=w294:T22)
            n137 = property on="Program step" class="LstBox (strict)"() -> ("Value"=w288:i32)  [unwired: 2 in, 2 out]
            n138 = Increment(x=w288) -> (x+1=w289:i32)
            n139 = Bundle By Name(cluster=w285, "Channel Type"="CAM", "Channels"=w278, "Wait/Poll (ms)"=w277, "Parameter"=w295) -> (w286:T20)
            n140 = Insert Into Array "Insert Into Array"(array=w294, index=w289, new element=w286) -> (w291:T22)
            n141 = Bundle By Name(cluster=w293, "Steps"=w291) -> (w292:T21)
            n142 = call "BuildStepListFromSteps.vi"("Steps"=w291, "Control Channels"=w282, "Feedback Channels"=w283, "AI"=w284) -> ("Step List"=w279:string[])  [unwired: 11 in]
            "Step List 4" <- w279
            n143 = Replace Array Subset(array=w281, new element=w292, index=w287) -> (w280:T4)
            n144 = property on="Program step" class="LstBox (strict)"("Key Focus"=TRUE, "Value"=w289, "Item Names"=w279) -> ()  [unwired: 2 in, 2 out]
          }
          frame True {
          }
        }
      }
      event "Analog": Value Change {
        n145 = event-data() -> ()  [unwired: 1 in, 1 out]
        n146 = property on="Feature List" class="MCListbox (strict)"() -> ("Value"=w302:i32)  [unwired: 2 in, 2 out]
        n147 = call "Configuration-PromptForChannelParameters_timer.vi"("Control/Feedback\n(Default: False = Feedback)"=FALSE ("Control/Feedback\n(Default: False = Feedback)")) -> ("Poll Time (Out)"=w322:u32, "Parameter (Out)"=w321:u8)  [unwired: 13 in]
        n148 = Select(t="AI", s="Analog", f="N") -> (s? t:f=w324:string)
        n149 = call "ConvertNumericChannelsToStringChannels.vi"("Channels (In)"="Analog Input") -> ("Channels (A:B:C:D...) (Out)"=w323:string)  [unwired: 14 in]
        n150 = property on="Program step" class="LstBox (strict)"() -> ("Value"=w312:i32)  [unwired: 2 in, 2 out]
        n151 = Bundle By Name(cluster=w318, "Channel Type"=w324, "Channels"=w323, "Wait/Poll (ms)"=w322, "Parameter"=w321) -> (w307:T20)
        n152 = Index Array(array=w311, index=w302) -> (element=w316:T21)
        n153 = Increment(x=w312) -> (x+1=w303:i32)
        n154 = Unbundle By Name(w316) -> ("Steps"=w317:T22)
        n155 = Insert Into Array(array=w317, index=w303, new element=w307) -> (w314:T22)
        n156 = Bundle By Name(cluster=w316, "Steps"=w314) -> (w315:T21)
        n157 = call "BuildStepListFromSteps.vi"("Steps"=w314, "Control Channels"=w308, "Feedback Channels"=w309, "AI"=w310) -> ("Step List"=w305:string[])  [unwired: 11 in]
        n158 = Replace Array Subset(array=w311, new element=w315, index=w302) -> (w306:T4)
        n159 = property on="Program step" class="LstBox (strict)"("Key Focus"=TRUE, "Value"=w303, "Item Names"=w305) -> ()  [unwired: 2 in, 2 out]
      }
      event Value Change {
        n160 = event-data() -> ()  [unwired: 1 in, 1 out]
        n161 = property on="Feature List" class="MCListbox (strict)"() -> ("Value"=w340:i32)  [unwired: 2 in, 2 out]
        n162 = property on="Program step" class="LstBox (strict)"() -> ("Value"=w339:i32)  [unwired: 2 in, 2 out]
        n163 = Select(t="STM", s="Motor", f="N") -> (s? t:f=w351:string)
        n164 = call "STM-program.vi"() -> ("OutDir"=w350:i32, "Out Speed"=w348:i32, "Out Degree"=w349:dbl, "Channels (A:B:C:D...) (Out)"=w328:string)  [unwired: 7 in, 1 out]
        n165 = Increment(x=w339) -> (x+1=w334:i32)
        n166 = Bundle By Name(cluster=w346, "Channel Type"=w351, "Channels"=w328, "Wait/Poll (ms)"=u32 0, "Parameter"=u8 0, "STM-Degree"=w349, "STM-Speed"=w348, "Direction"=w350) -> (w331:T20)
        n167 = Index Array(array=w341, index=w340) -> (element=w344:T21)
        n168 = Unbundle By Name(w344) -> ("Steps"=w345:T22)
        n169 = Insert Into Array(array=w345, index=w334, new element=w331) -> (w342:T22)
        n170 = Bundle By Name(cluster=w344, "Steps"=w342) -> (w343:T21)
        n171 = local write "Motor"(FALSE ("Motor")) -> ()
        n172 = call "BuildStepListFromSteps.vi"("Steps"=w342, "Control Channels"=w338, "Feedback Channels"=w337, "AI"=w336) -> ("Step List"=w332:string[])  [unwired: 11 in]
        n173 = Replace Array Subset(array=w341, new element=w343, index=w340) -> (w333:T4)
        n174 = property on="Program step" class="LstBox (strict)"("Key Focus"=TRUE, "Value"=w334, "Item Names"=w332) -> ()  [unwired: 2 in, 2 out]
      }
      event Value Change {
        n175 = event-data() -> ()  [unwired: 1 in, 1 out]
        n176 = property on="Feature List" class="MCListbox (strict)"() -> ("Value"=w354:i32)  [unwired: 2 in, 2 out]
        n177 = Index Array(array=w362, index=w354) -> (element=w365:T21)
        n178 = Bundle By Name(cluster=w371, "Channel Type"="N", "Wait/Poll (ms)"="Wait Time") -> (w367:T20)
        n179 = Unbundle By Name(w365) -> ("Steps"=w366:T22)
        n180 = property on="Program step" class="LstBox (strict)"() -> ("Value"=w368:i32)  [unwired: 2 in, 2 out]
        n181 = Increment(x=w368) -> (x+1=w355:i32)
        n182 = Insert Into Array(array=w366, index=w355, new element=w367) -> (w363:T22)
        n183 = Bundle By Name(cluster=w365, "Steps"=w363) -> (w364:T21)
        n184 = call "BuildStepListFromSteps.vi"("Steps"=w363, "Control Channels"=w360, "Feedback Channels"=w359, "AI"=w357) -> ("Step List"=w358:string[])  [unwired: 11 in]
        n185 = property on="Program step" class="LstBox (strict)"("Item Names"=w358, "Value"=w355, "Key Focus"=TRUE) -> ()  [unwired: 2 in, 2 out]
        n186 = Replace Array Subset(array=w362, new element=w364, index=w354) -> (w361:T4)
      }
      event Value Change {
        n187 = event-data() -> ()  [unwired: 1 in, 2 out]
        n188 = property on="Feature List" class="MCListbox (strict)"() -> ("Value"=w373:i32)  [unwired: 2 in, 2 out]
        n189 = Index Array(array=w384, index=w373) -> (element=w390:T21)
        n190 = property on="Program step" class="LstBox (strict)"() -> ("Value"=w372:i32)  [unwired: 2 in, 2 out]
        n191 = Unbundle By Name(w390) -> ("Item Name"=w388:string, "Item Status"=w387:bool, "Steps"=w386:T22)
        n192 = Equal?(x=w372, y=-1) -> (x = y?=w376:bool)
        n193 = Select(t=0 ("y"), s=w376, f=w372) -> (s? t:f=w374:i32)
        n194 = Delete From Array(array=w386, length=1, index=w374) -> (array with subset deleted=w382:T22)  [unwired: 1 out]
        n195 = Bundle("Item Name"=w388, "Item Status"=w387, "Steps"=w382) -> (w385:T21)  [unwired: 1 in]
        n196 = call "BuildStepListFromSteps.vi"("Steps"=w382, "Control Channels"=w380, "Feedback Channels"=w379) -> ("Step List"=w378:string[])  [unwired: 12 in]
        n197 = Replace Array Subset(array=w384, new element=w385, index=w373) -> (w383:T4)
        n198 = property on="Program step" class="LstBox (strict)"("Item Names"=w378, "Value"=w374, "Key Focus"=TRUE) -> ()  [unwired: 2 in, 2 out]
      }
      event Value Change {
        n199 = event-data() -> ()  [unwired: 1 in, 1 out]
        n200 = for {
          tunnel: w393 -> [w440] mode=indexing
          tunnel: [w435] -> w401 mode=indexing
          shift-right: [w434] -> w402
          shift-left: w409 -> [w437]
          n201 = Unbundle By Name(w440) -> ("Steps"=w441:T22, "Item Name"=w439:string, "Item Status"=w438:bool)
          n202 = Array Size(array=w441) -> (size(s)=w436:i32)
          n203 = case shown="Default" w436 {
            tunnel: w441 -> [_ w448]
            tunnel: w439 -> [_ w450]
            tunnel: w438 -> [_ w449]
            tunnel: [w443 w446] -> w434
            tunnel: w437 -> [w443 w444]
            tunnel: [FALSE TRUE] -> w435
            frame 0 {
            }
            frame Default {
              n204 = Bundle("Item Name"=w450, "Item Status"=w449, "Steps"=w448) -> (w445:T21)  [unwired: 1 in]
              n205 = Build Array (concatenate)(w444, w445) -> (w446:T4)
            }
          }
        }
        n206 = And Array Elements(Boolean array=w401) -> (logical AND=w400:bool)
        n207 = case shown="True" w400 {
          tunnel: [w413 w415] -> w395
          tunnel: w394 -> [_ w423]
          tunnel: [_ w421] -> w403
          tunnel: w402 -> [_ w416]
          tunnel: enum16{"Read", "Write"}."Write" ("Read/Write") -> [_ w422]
          tunnel: "Feature List successfully saved." -> [_ w420]
          tunnel: "Error in saving Feature List." -> [_ w419]
          tunnel: "Can't save Feature List as at least one feature doesn't have steps.\nPlease check." ("message") -> [w414 w418]
          tunnel: w393 -> [w413 _]
          frame False {
            n208 = One Button Dialog(message=w414) -> ()  [unwired: 1 in, 1 out]
          }
          frame True {
            n209 = call "FileIO-ReadWrite-FeatureList.vi"("Filepath"=w423, "Feature List (In)"=w416, "Read/Write"=w422) -> ("Feature List (Out)"=w415:T4, "Error Out"=w421:errorcluster)  [unwired: 11 in]
            n210 = case shown="Error" w421 {
              tunnel: w420 -> [w424 _]
              tunnel: w419 -> [_ w425]
              tunnel: w418 -> [_ _]
              tunnel: [w424 w425] -> w417
              frame No Error {
              }
              frame Error {
              }
            }
            n211 = One Button Dialog(message=w417) -> ()  [unwired: 1 in, 1 out]
          }
        }
        n212 = disable-structure shown="Enabled" {
          frame Disabled {
            n213 = call "Program seq path.vi"() -> ()  [unwired: 11 in, 1 out]
          }
          frame Enabled {
          }
        }
        n214 = Index Array(array=w395, index=0) -> (element=w407:T21)
        n215 = Unbundle By Name(w407) -> ("Steps"=w406:T22)
        n216 = for {
          tunnel: [w432] -> w392 mode=indexing
          tunnel: w395 -> [w427] mode=indexing
          tunnel: [w426] -> _
          i -> [w426]
          n217 = Unbundle By Name(w427) -> ("Item Name"=w433:string, "Item Status"=w431:bool)
          n218 = Select(t="Active", s=w431, f="Inactive") -> (s? t:f=w428:string)
          n219 = Build Array(w433, w428) -> (w432:string[])
        }
        n220 = call "BuildStepListFromSteps.vi"("Steps"=w406, "Control Channels"=w412, "Feedback Channels"=w411, "AI"=w404) -> ("Step List"=w410:string[])  [unwired: 11 in]
        n221 = property on="Program step" class="LstBox (strict)"("Item Names"=w410, "Value"=0 ("Step feautre list")) -> ()  [unwired: 2 in, 2 out]
        n222 = property on="Feature List" class="MCListbox (strict)"("ItemNames"=w392, "Value"=0 ("Feautre list")) -> ()  [unwired: 2 in, 2 out]
      }
      event Value Change {
        n223 = event-data() -> ()  [unwired: 1 in, 1 out]
      }
      event "Program step": Double Click {
        n224 = event-data() -> ("Row"=w467:i32)  [unwired: 1 in, 8 out]
        n225 = property on="Program step" class="LstBox (strict)"() -> ("Item Names"=w468:string[])  [unwired: 2 in, 2 out]
        n226 = Index Array(array=w468, index=w467) -> (element=w458:string)
        n227 = String Length(string=w458) -> (length=w457:i32)
        n228 = String Subset(string=w458, length (rest)=2 ("length (rest)")) -> (substring=w463:string)  [unwired: 1 in]
        n229 = String Subset(string=w458, length (rest)=4 ("length (rest)")) -> (substring=w461:string)  [unwired: 1 in]
        n230 = Less Or Equal?(x=w457, y=0) -> (x <= y?=w454:bool)
        "x <= y?" <- w454
        n231 = Equal?(x=w461, y="Wait") -> (x = y?=w459:bool)
        n232 = Equal?(x=w463, y="Ch") -> (x = y?=w464:bool)
        n233 = case shown="False" w454 {
          tunnel: w476 -> [w487 _]
          tunnel: w475 -> [w486 w550]
          tunnel: w474 -> [w485 _]
          tunnel: w473 -> [w484 _]
          tunnel: w472 -> [w483 _]
          tunnel: [w482 w550] -> w471
          tunnel: [w481 w551] -> w470
          tunnel: w469 -> [w480 w551]
          tunnel: w464 -> [w479 _]
          tunnel: w459 -> [w478 _]
          tunnel: enum32{"Output", "Input"}."Output" ("y") -> [w477 _]
          frame False {
            n234 = case shown="False" w478 {
              tunnel: w487 -> [w504 w537]
              tunnel: w486 -> [w503 w536]
              tunnel: w485 -> [w502 w540]
              tunnel: w484 -> [w501 w539]
              tunnel: w483 -> [w500 w538]
              tunnel: [w499 w535] -> w482
              tunnel: [w498 w534] -> w481
              tunnel: w480 -> [w492 _]
              tunnel: w479 -> [w491 _]
              tunnel: w477 -> [w489 _]
              frame False {
                n235 = call "DO Control.vi"("s"=w491) -> ("Feedback"=w494:i32[], "Parameter (Out)"=w495:u8, "Control Channel"=w497:i32[], "Poll Time (Out)"=w496:u32, "Tab Control 2"=w488:enum32{"Output", "Input"}, "Cancel"=w490:bool)  [unwired: 5 in]
                n236 = Equal?(x=w488, y=w489) -> (x = y?=w493:bool)
                n237 = case shown="False" w490 {
                  tunnel: w504 -> [w529 _]
                  tunnel: w503 -> [w528 w531]
                  tunnel: w502 -> [w527 _]
                  tunnel: w501 -> [w526 _]
                  tunnel: w500 -> [w525 _]
                  tunnel: [w524 w531] -> w499
                  tunnel: [w523 w532] -> w498
                  tunnel: w497 -> [w514 _]
                  tunnel: w496 -> [w513 _]
                  tunnel: w495 -> [w512 _]
                  tunnel: w494 -> [w511 _]
                  tunnel: w493 -> [w505 _]
                  tunnel: w492 -> [_ w532]
                  frame False {
                    n238 = property on="Feature List" class="MCListbox (strict)"() -> ("Value"=w515:i32)  [unwired: 2 in, 2 out]
                    n239 = Index Array(array=w528, index=w515) -> (element=w520:T21)
                    n240 = Select(t="C", s=w505, f="F") -> (s? t:f=w508:string)
                    n241 = Select(t=w514, s=w505, f=w511) -> (s? t:f=w507:i32[])
                    n242 = disable-structure shown="Disabled" {
                      disable-tunnel: w505 -> [w530 _]
                      frame Disabled {
                        n243 = call "Configuration-PromptForChannelParameters_timer.vi"("Control/Feedback\n(Default: False = Feedback)"=w530) -> ()  [unwired: 13 in, 2 out]
                      }
                      frame Enabled {
                      }
                    }
                    n244 = call "ConvertNumericChannelsToStringChannels.vi"("Channels (In)"=w507) -> ("Channels (A:B:C:D...) (Out)"=w506:string)  [unwired: 14 in]
                    n245 = Unbundle By Name(w520) -> ("Steps"=w522:T22)
                    n246 = Bundle By Name(cluster=w529, "Channel Type"=w508, "Channels"=w506, "Wait/Poll (ms)"=w513, "Parameter"=w512) -> (w521:T20)
                    n247 = property on="Program step" class="LstBox (strict)"() -> ("Value"=w516:i32)  [unwired: 2 in, 2 out]
                    n248 = Replace Array Subset(array=w522, new element=w521, index=w516) -> (w518:T22)
                    n249 = Bundle By Name(cluster=w520, "Steps"=w518) -> (w519:T21)
                    n250 = call "BuildStepListFromSteps.vi"("Steps"=w518, "Control Channels"=w525, "Feedback Channels"=w526, "AI"=w527) -> ("Step List"=w523:string[])  [unwired: 11 in]
                    "Step List 2" <- w523
                    n251 = Replace Array Subset(array=w528, new element=w519, index=w515) -> (w524:T4)
                    n252 = property on="Program step" class="LstBox (strict)"("Key Focus"=TRUE, "Value"=w516, "Item Names"=w523) -> ()  [unwired: 2 in, 2 out]
                  }
                  frame True {
                  }
                }
              }
              frame True {
                n253 = property on="Feature List" class="MCListbox (strict)"() -> ("Value"=w541:i32)  [unwired: 2 in, 2 out]
                n254 = call "Timer.vi"() -> ("Wait Time out"=w533:u32)  [unwired: 10 in, 1 out]
                n255 = Index Array(array=w536, index=w541) -> (element=w545:T21)
                n256 = Bundle By Name(cluster=w537, "Channel Type"="N", "Wait/Poll (ms)"=w533) -> (w547:T20)
                n257 = Unbundle By Name(w545) -> ("Steps"=w546:T22)
                n258 = property on="Program step" class="LstBox (strict)"() -> ("Value"=w548:i32)  [unwired: 2 in, 2 out]
                n259 = Replace Array Subset(array=w546, new element=w547, index=w548) -> (w543:T22)
                n260 = Bundle By Name(cluster=w545, "Steps"=w543) -> (w544:T21)
                n261 = call "BuildStepListFromSteps.vi"("Steps"=w543, "Control Channels"=w538, "Feedback Channels"=w539, "AI"=w540) -> ("Step List"=w534:string[])  [unwired: 11 in]
                n262 = property on="Program step" class="LstBox (strict)"("Item Names"=w534, "Value"=w548, "Key Focus"=TRUE) -> ()  [unwired: 2 in, 2 out]
                n263 = Replace Array Subset(array=w536, new element=w544, index=w541) -> (w535:T4)
              }
            }
          }
          frame True {
          }
        }
      }
      event Panel Close? {
        n264 = event-data() -> ()  [unwired: 1 in, 1 out]
        n265 = event-data("Discard?"=TRUE) -> ()  [unwired: 1 in, 1 out]
      }
    }
  }
  "Error Out" <- w23
